vi "item name2.vi"() -> ()   [LabVIEW 2020]
panel:
  in  "Item Name2":string[](array[string])
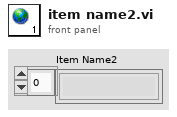
[diagram p1: front panel]
diagram:
